vi "Save-Load PhXP Settings.vi"(6 "Load(F)/Save (T)":bool, 8 "Error In":errorcluster, 10 "File Path":path) -> (0 "Error Out":errorcluster, 2 "File Path out":path)   [LabVIEW 2019]
doc: "Use this file to Save or Load AlliGator's settings to an ini file.\nIf the Path input is left unconnected, the defaut ini file is used (overriding the current ini file).\nTo save settings in a user-specified location, either provide a valid path, or connect a \"Not a Path\" constant to the input. A File Dialog window will then open to allow the user to choose a path."
uses:
  Phasor Explorer Settings List.ctl
  <vilib>/Utility/sysdir.llb/System Directory Type.ctl
  <vilib>/Utility/config.llb/NI_LVConfig.lvlib
panel:
  in  "PhXP Settings List":T1
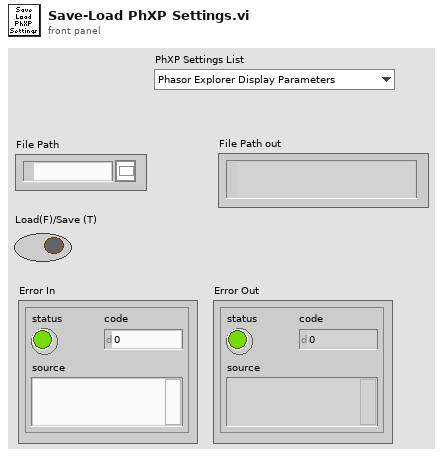
[diagram p1: front panel]
types:
  T1 = typedef "Phasor Explorer Settings List.ctl" = enum16{"Phasor Explorer Display Parameters", "Phasor Explorer Phasor Parameters", "Phasor Explorer Decay & IRF Parameters", "Phasor Explorer Gate Parameters", "Phasor Explorer Detector Parameters", "f*", "tau*"}
  T2 = typedef "System Directory Type.ctl" = i32
  T3 = typedef "NI_LVConfig.lvlib/Config Data RefNum.ctl" = refnum<k1>
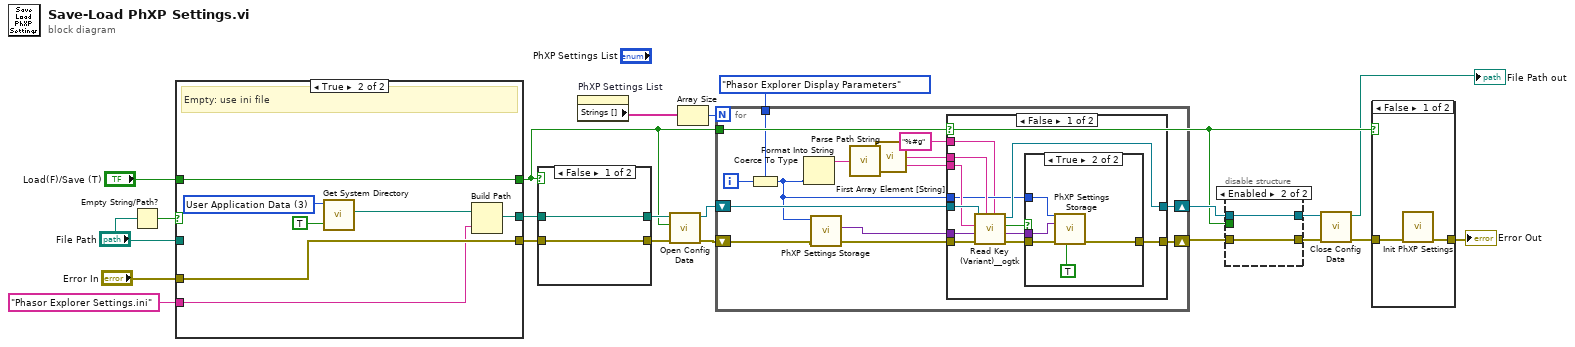
[diagram p0: block diagram]
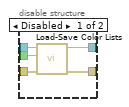
[diagram p3: hidden frame]
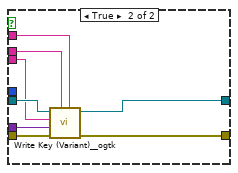
[diagram p5: hidden frame]
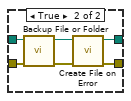
[diagram p6: hidden frame]
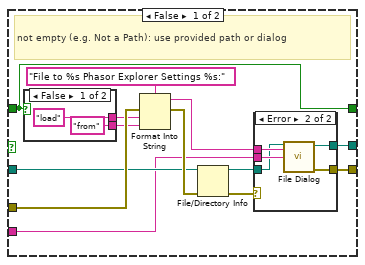
[diagram p7: hidden frame]
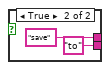
[diagram p9: hidden frame]
diagram:
  n1 = Empty String/Path?(string/path="File Path") -> (empty?=w9:bool)
  n2 = case shown="True" w9 {
    tunnel: [w35 w50] -> w22
    tunnel: "Error In" -> [w31 w49]
    tunnel: [w34 w49] -> w7
    tunnel: "File Path" -> [w25 _]
    tunnel: "Load(F)/Save (T)" -> [w28 w48]
    tunnel: [w28 w48] -> w4
    tunnel: "Phasor Explorer Settings.ini" ("name or relative path") -> [w23 w47]
    frame False {
      # "not empty (e.g. Not a Path): use provided path or dialog"
      n3 = case shown="False" w28 {
        tunnel: ["load" ("input 1") "save" ("input 1")] -> w30
        tunnel: ["from" ("input 2") "to" ("input 2")] -> w29
        frame False {
        }
        frame True {
        }
      }
      n4 = Format Into String(format string="File to %s Phasor Explorer Settings %s:" ("prompt"), error in=w31, w30, w29) -> (resulting string=w32:string, error out=w27:errorcluster)  [unwired: 1 in]
      n5 = File/Directory Info(path=w25, error in=w27) -> (path out=w24:path, error out=w26:errorcluster)  [unwired: 5 out]
      n6 = case shown="Error" w26 {
        selector: w26 -> [w36 _]
        tunnel: [w37 w42] -> w35
        tunnel: [w36 w41] -> w34
        tunnel: w23 -> [_ w40]
        tunnel: w32 -> [_ w39]
        tunnel: w24 -> [w37 w38]
        frame No Error {
        }
        frame Error {
          n7 = call "File Dialog"("start path"=w38, "prompt"=w39, "default name"=w40) -> ("selected path"=w42:path, "error out"=w41:errorcluster)  [unwired: 9 in, 2 out]
        }
      }
    }
    frame True {
      w51 = T2 3 items=["User Home"=0, "User Desktop"=1, "User Documents"=2, "User Application Data"=3, "User Preferences"=4, "User Temporary"=5, "Public Documents"=6, "Public Application Data"=7, "Public Preferences"=8, "Public Cache"=13, "System Core Libraries"=9, "System Installed Libraries"=10, "Application Files"=11, "Boot Volume Root"=12] ("system directory type")
      # "Empty: use ini file"
      n8 = call <vilib>:"Get System Directory.vi"("create directory if not found? (F)"=TRUE, "system directory type"=w51) -> ("system directory"=w52:path)  [unwired: 9 in]
      n9 = Build Path(base path=w52, name or relative path=w47) -> (appended path=w50:path)
    }
  }
  n10 = case shown="False" w4 {
    tunnel: w22 -> [w55 w61]
    tunnel: w7 -> [w54 w60]
    tunnel: [w55 w57] -> w21
    tunnel: [w54 w56] -> w20
    frame False {
    }
    frame True {
      n11 = call "Backup File or Folder.vi"("error in (no error)"=w60, "File/Directory Path"=w61) -> ("error out"=w58:errorcluster, "File/Directory Path (dup)"=w59:path)  [unwired: 8 in]
      n12 = call "Create File on Error.vi"("error in (no error)"=w58, "File Path"=w59) -> ("error out"=w56:errorcluster, "File Path (dup)"=w57:path)  [unwired: 8 in]
    }
  }
  n13 = property on="PhXP Settings List" class="Enum (strict)"() -> ("Strings []"=w16:string[])  [unwired: 2 in, 2 out]
  n14 = call <vilib>:"Open Config Data.vi"("error in (no error)"=w20, "create file if necessary (T)"=w4, "configuration file path"=w21) -> ("error out"=w19:errorcluster, "refnum"=w18:T3)  [unwired: 6 in, 1 out]
  n15 = Array Size(array=w16) -> (size(s)=w15:i32)
  n16 = for {
    N: w15 -> [_]
    shift-right: [w71] -> w12
    shift-left: w19 -> [w64]
    shift-right: [w72] -> w13
    shift-left: w18 -> [w73]
    tunnel: Phasor_Explorer_Settings_List."Phasor Explorer Display Parameters" ("PhXP Settings List") -> [w75]
    tunnel: w4 -> [w74]
    i -> [w76]
    n17 = Coerce To Type(0:w76, 1:w75) -> (2:w65:T1)
    n18 = Format Into String(w65) -> (resulting string=w70:string)  [unwired: 3 in, 1 out]
    n19 = call "PhXP Settings Storage.vi"("Error In"=w64, "Settings List"=w65) -> ("Error Out"=w62:errorcluster, "Variant Data out"=w63:variant)  [unwired: 8 in]
    n20 = call "Parse Path String.vi"("Path in"=w70) -> ("Folder Hierarchy"=w68:string[], "File/Folder"=w69:string)  [unwired: 4 in]
    n21 = call "First Array Element [String].vi"("Array"=w68) -> ("First Element"=w67:string)  [unwired: 8 in]
    n22 = case shown="False" w74 {
      tunnel: w73 -> [w88 w102]
      tunnel: [w85 w101] -> w72
      tunnel: w63 -> [w87 w98]
      tunnel: w62 -> [w86 w100]
      tunnel: [w81 w99] -> w71
      tunnel: w69 -> [w84 w97]
      tunnel: w67 -> [w83 w96]
      tunnel: w65 -> [w80 _]
      tunnel: "%#g" ("float number format") -> [w77 w95]
      frame False {
        n23 = call <userlib>:"Read Key (Variant)__ogtk.vi"("format string (%;%f)"=w77, "section"=w83, "error in (no error)"=w86, "type"=w87, "key (optional)"=w84, "refnum"=w88) -> ("error out"=w82:errorcluster, "key-value"=w79:variant, "found?"=w78:bool, "refnum out"=w85:T3)  [unwired: 2 in]
        n24 = case shown="True" w78 {
          tunnel: w82 -> [w89 w94]
          tunnel: [w89 w90] -> w81
          tunnel: w80 -> [_ w91]
          tunnel: w79 -> [_ w92]
          frame False {
          }
          frame True {
            n25 = call "PhXP Settings Storage.vi"("Set/Get(F)"=TRUE ("Get (F)/Set"), "Error In"=w94, "Variant Data in"=w92, "Settings List"=w91) -> ("Error Out"=w90:errorcluster)  [unwired: 6 in, 1 out]
          }
        }
      }
      frame True {
        n26 = call <userlib>:"Write Key (Variant)__ogtk.vi"("float number format"=w95, "section"=w96, "error in (no error)"=w100, "key-value"=w98, "key (optional)"=w97, "refnum"=w102) -> ("error out"=w99:errorcluster, "refnum out"=w101:T3)  [unwired: 4 in]
      }
    }
  }
  n27 = disable-structure shown="Enabled" {
    disable-tunnel: w13 -> [w107 w109]
    disable-tunnel: w12 -> [w106 w108]
    disable-tunnel: [w105 w109] -> w11
    disable-tunnel: [w104 w108] -> w10
    disable-tunnel: w4 -> [w103 _]
    frame Disabled {
      n28 = call "Load-Save Color Lists.vi"("error in (no error)"=w106, "Load (F)/Save"=w103, "ini File Refnum in"=w107) -> ("error out"=w104:errorcluster, "ini File Refnum out"=w105:T3)  [unwired: 7 in]
    }
    frame Enabled {
    }
  }
  n29 = call <vilib>:"Close Config Data.vi"("error in (no error)"=w10, "refnum"=w11) -> ("error out"=w17:errorcluster, "file path"=→"File Path out":path)  [unwired: 8 in]
  n30 = case shown="False" w4 {
    tunnel: w17 -> [w111 w112]
    tunnel: [w110 w112] -> w14
    frame False {
      n31 = call "Init PhXP Settings.vi"("error in (no error)"=w111) -> ("error out"=w110:errorcluster)  [unwired: 10 in]
    }
    frame True {
    }
  }
  "Error Out" <- w14
